vi "SUB_READ_KT300WR2_IPEI_UUT.vi"(5 "VISA resource name":refnum<visa-resource-name>) -> (0 "debug View":string, 1 "UUT_IPEI":string, 2 "Found IPEI ?":bool)   [LabVIEW 2011]
panel:
  out "length":i32
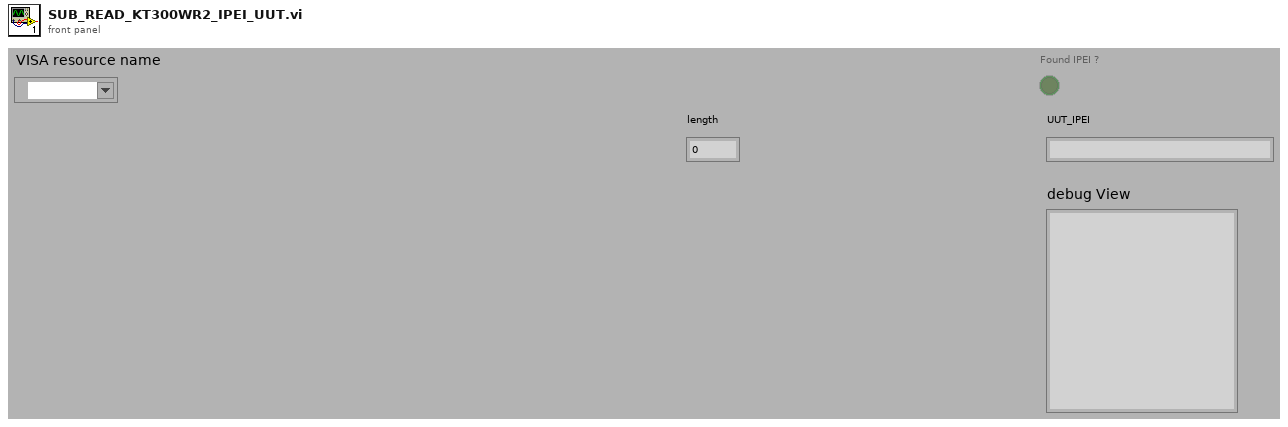
[diagram p1: front panel]
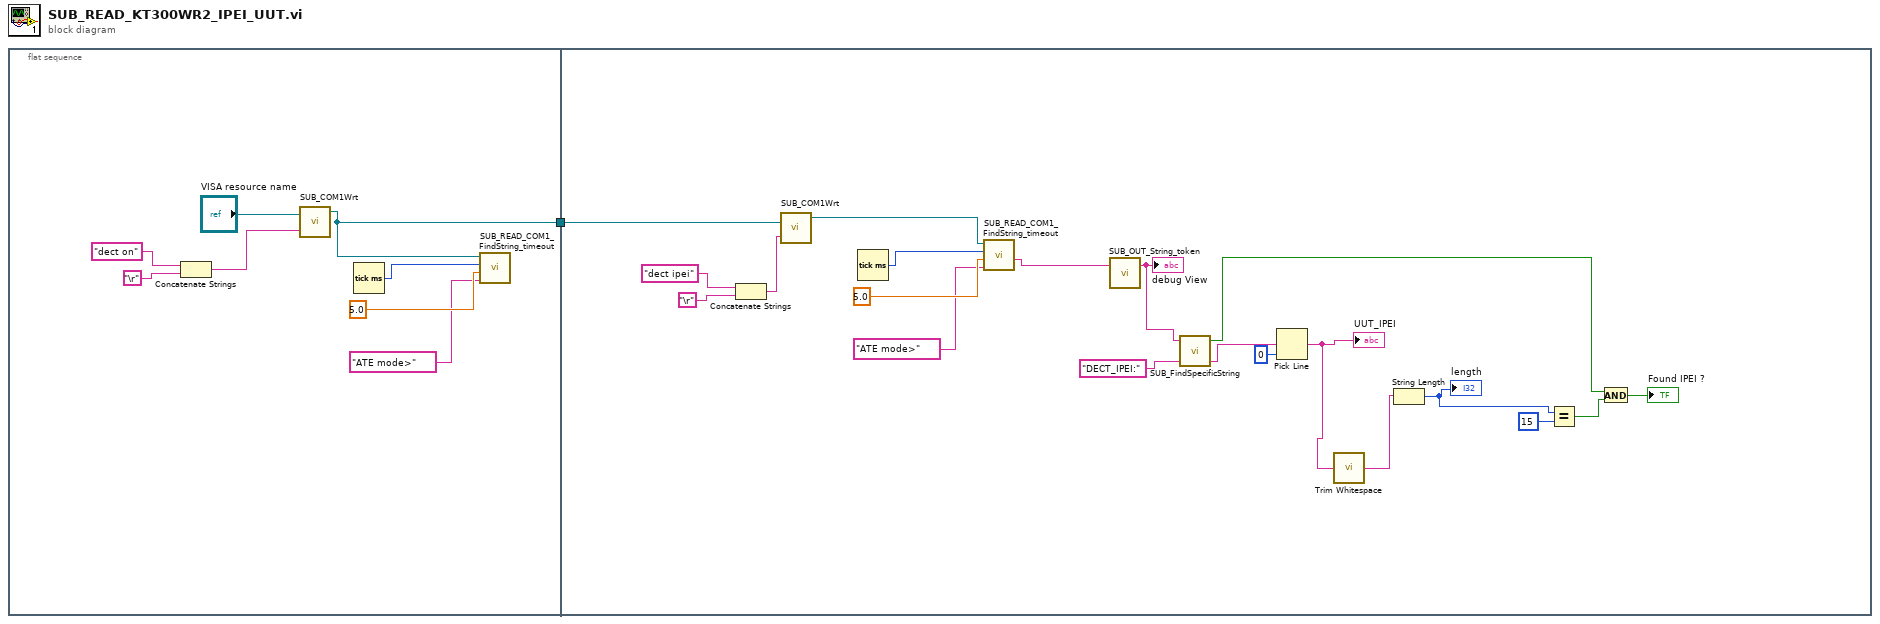
[diagram p0: block diagram]
diagram:
  n1 = flat-sequence {
    tunnel: [w3] -> w1
    tunnel: w1 -> [w26]
    frame #0 {
      n2 = Concatenate Strings("dect on" ("string"), "\r") -> (w7:string)
      n3 = call "SUB_COM1Wrt.vi"("VISA resource name"="VISA resource name", "write buffer"=w7) -> ("duplicate VISA resource name"=w3:refnum<visa-resource-name>)  [unwired: 2 out]
      n4 = Tick Count (ms)() -> (millisecond timer value=w6:u32)
      n5 = call "SUB_READ_COM1_FindString_timeout.vi"("Find this String"="ATE mode>", "Timeout Seccond"=5.0, "Begin time"=w6, "duplicate VISA resource name 2"=w3) -> ()  [unwired: 1 in, 3 out]
    }
    frame #1 {
      n6 = Concatenate Strings("dect ipei" ("string"), "\r") -> (w29:string)
      n7 = call "SUB_COM1Wrt.vi"("VISA resource name"=w26, "write buffer"=w29) -> ("duplicate VISA resource name"=w23:refnum<visa-resource-name>)  [unwired: 2 out]
      n8 = Tick Count (ms)() -> (millisecond timer value=w25:u32)
      n9 = call "SUB_READ_COM1_FindString_timeout.vi"("Find this String"="ATE mode>", "Timeout Seccond"=5.0, "Begin time"=w25, "duplicate VISA resource name 2"=w23) -> ("Output String"=w21:string)  [unwired: 1 in, 2 out]
      n10 = call "SUB_OUT_String_token.vi"("input string"=w21) -> ("result string"=w19:string)  [unwired: 2 in]
      "debug View" <- w19
      n11 = call "SUB_FindSpecificString.vi"("Find this String"="DECT_IPEI:", "String data"=w19) -> ("before \"; \" string"=w18:string, "Found"=w11:bool)  [unwired: 2 in]
      n12 = Pick Line(multi-line string=w18, line index=0) -> (output string=w16:string)  [unwired: 1 in]
      "UUT_IPEI" <- w16
      n13 = call <vilib>:"Trim Whitespace.vi"("string"=w16) -> ("trimmed string"=w15:string)  [unwired: 1 in]
      n14 = String Length(string=w15) -> (length=w14:i32)
      "length" <- w14
      n15 = Equal?(x=w14, y=15) -> (x = y?=w12:bool)
      n16 = And(x=w11, y=w12) -> (x .and. y?=→"Found IPEI ?":bool)
    }
  }
